vi "Additional Results.vi"(8 "error in (no error)":errorcluster, 9 "Sequenc Context":refnum<class "Configuration.lvclass">, 10 "Array in":string[](array[string]), 11 "TestStand Result Handler in":refnum<class "TestStand Result Handler.lvclass">) -> (0 "error out":errorcluster, 2 "Array":string[](array[string]), 3 "TestStand Result Handler out":refnum<class "TestStand Result Handler.lvclass">)   [LabVIEW 2020, in "Astemes_CSVReportPlugin.lvlib" / "TestStand Result Handler.lvclass"]
doc: "Template method called before adding the result to the report. Use this to add additional results to the report by adding them to the array."
uses:
  TestStand Result Handler.lvclass
  Configuration/Configuration.lvclass
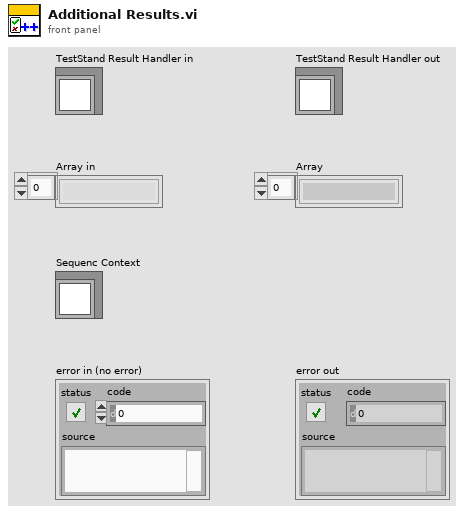
[diagram p1: front panel]
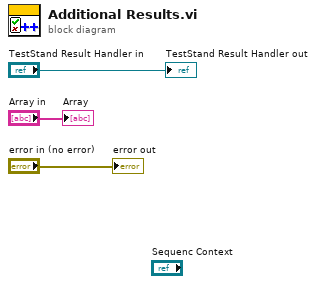
[diagram p0: block diagram]
diagram:
  "Array" <- "Array in"
  "error out" <- "error in (no error)"
  "TestStand Result Handler out" <- "TestStand Result Handler in"
